vi "Configure Trigger (TV).vi"(0 "VISA resource name":refnum<visa-resource-name>, 2 "Trigger Source (1: Channel 1)":u16(ring)=1 items=["Channel 1"=1, "Channel 2"=2, "Channel 3"=3, "Channel 4"=4, "Ext"=5, "Ext5"=6], 9 "Characteristic (0: NTSC)":u16(ring) items=["NTSC", "Pal/Secam"], 11 "error in (no error)":errorcluster, 12 "Sync (0: All Lines)":u16(ring) items=["All Lines", "Line Num", "Odd Field", "Even Field"], 13 "Line Num (200)":dbl=200.0) -> (4 "VISA resource name out":refnum<visa-resource-name>, 15 "error out":errorcluster)   [LabVIEW 2021, in "Siglent SDS 1000 2000 Series.lvlib"]
doc: "Configures TV triggers that provide stable triggering on standard or custom composite video signals. Use them on Pal/Secam or NTSC systems. A composite video signal on the trigger input is analyzed to provide a signal for the beginning of the chosen field and for a signal at the beginning of each line. The field signal provides the starting transition, and the beginnings of line pulses are counted to allow the final trigger on the chosen line. For each field, the number of fields, the field rate, interlace factor, and number of lines per picture must be specified although there are standard settings for the most common types of TV signals. TV Trigger can also function in a simple any-line mode."
uses:
  <instrlib>/Siglent SDS 1000 2000 Series/Siglent SDS 1000 2000 Series.lvlib
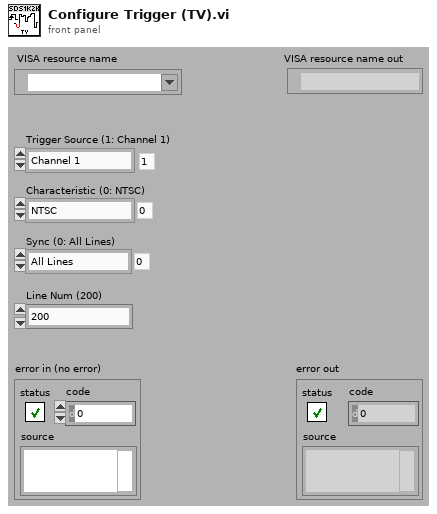
[diagram p1: front panel]
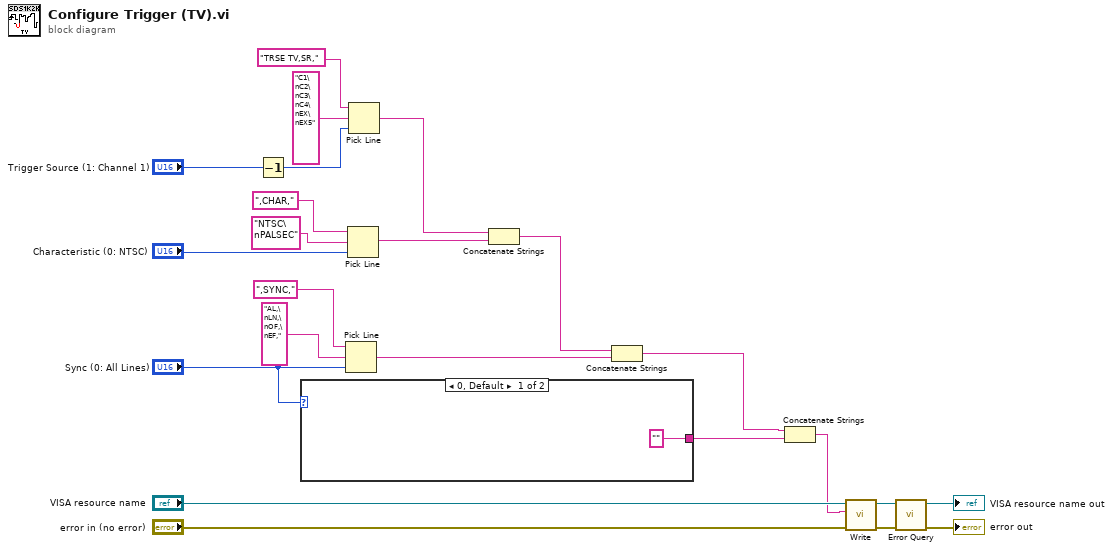
[diagram p0: block diagram]
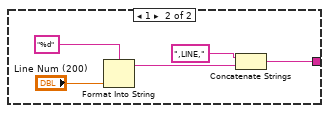
[diagram p2: hidden frame]
diagram:
  n1 = Decrement(x="Trigger Source (1: Channel 1)") -> (x-1=w1:u16)
  n2 = case shown="0, Default" "Sync (0: All Lines)" {
    tunnel: ["" w26] -> w5
    frame 0, Default {
    }
    frame 1 {
      n3 = Format Into String(format string="%d", "Line Num (200)") -> (resulting string=w29:string)  [unwired: 2 in, 1 out]
      n4 = Concatenate Strings(",LINE," ("string"), w29) -> (w26:string)
    }
  }
  n5 = Pick Line(string ("")=",SYNC,", multi-line string="AL,\nLN,\nOF,\nEF,", line index="Sync (0: All Lines)") -> (output string=w11:string)
  n6 = Pick Line(string ("")=",CHAR,", multi-line string="NTSC\nPALSEC", line index="Characteristic (0: NTSC)") -> (output string=w9:string)
  n7 = Pick Line(string ("")="TRSE TV,SR,", multi-line string="C1\nC2\nC3\nC4\nEX\nEX5", line index=w1) -> (output string=w13:string)
  n8 = Concatenate Strings(w13, w9) -> (w14:string)
  n9 = Concatenate Strings(w14, w11) -> (w4:string)
  n10 = Concatenate Strings(w4, w5) -> (w3:string)
  n11 = call <instrlib>:"Write.vi"("error in (no error)"="error in (no error)", "Write Buffer"=w3, "VISA resource name"="VISA resource name") -> ("error out"=w20:errorcluster, "VISA resource name out"=w21:refnum<visa-resource-name>)  [unwired: 6 in, 1 out]
  n12 = call <instrlib>:"Error Query.vi"("error in (no error)"=w20, "VISA resource name"=w21) -> ("error out"=→"error out":errorcluster, "VISA resource name out"=→"VISA resource name out":refnum<visa-resource-name>)  [unwired: 6 in, 2 out]
